vi "DotProduct.vi"(1 "Y":T1, 2 "X":T1) -> (0 "X*Y":dbl)   [LabVIEW 2017, in "ArgosLib.lvlib"]
uses:
  ArgosLib.lvlib
  Path Planning/TypeDefs/Point2D.ctl
  <vilib>/Analysis/baseanly.llb/Real Dot Product.vi
  <vilib>/Analysis/NI_AALBase.lvlib
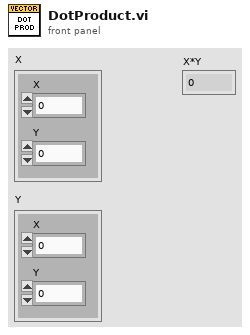
[diagram p1: front panel]
types:
  T1 = typedef "ArgosLib.lvlib/Point2D.ctl" = cluster{"X":dbl, "Y":dbl}
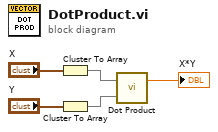
[diagram p0: block diagram]
diagram:
  n1 = Cluster To Array(cluster="X") -> (array=w3:dbl[])
  n2 = Cluster To Array(cluster="Y") -> (array=w2:dbl[])
  n3 = call-poly <vilib>:"Dot Product.vi"("Y Vector"=w2, "X Vector"=w3) -> ("X * Y"=→"X*Y":dbl)  [unwired: 1 out]
